vi "WriteDoubleGlobal.vi"(0 "controller in":refnum<k24>, 7 "variable number":i32, 9 "value":dbl, 11 "error in (no error)":errorcluster) -> (4 "controller out":refnum<k24>, 15 "error out":errorcluster)   [LabVIEW 2019]
uses:
  C:/Users/patrick/Documents/GitHub/Aerotech-Delay-Line/lvsrc/Aerotech-Ensemble-LabVIEW/2010-5.6/Bin/Aerotech.Ensemble.dll
  Bin/Aerotech.Ensemble.dll
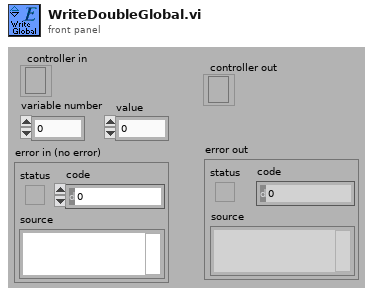
[diagram p1: front panel]
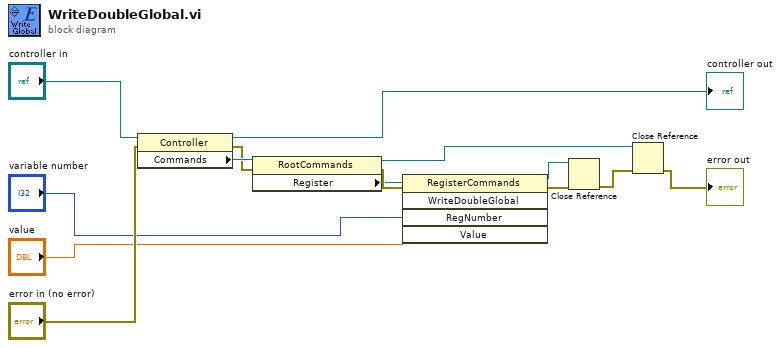
[diagram p0: block diagram]
diagram:
  n1 = property class="Controller"(reference="controller in", error in="error in (no error)") -> (reference out=→"controller out":refnum<k24>, error out=w10:errorcluster, "Commands"=w11:refnum<k24>)
  n2 = property class="RootCommands"(reference=w11, error in=w10) -> (reference out=w3:refnum<k24>, error out=w9:errorcluster, "Register"=w8:refnum<k24>)
  n3 = invoke class="RegisterCommands" method="WriteDoubleGlobal"(reference=w8, error in=w9, "RegNumber"="variable number", "Value"="value") -> (reference out=w4:refnum<k24>, error out=w7:errorcluster)  [unwired: 1 in, 3 out]
  n4 = Close Reference(reference=w4, error in (no error)=w7) -> (error out=w5:errorcluster)
  n5 = Close Reference(reference=w3, error in (no error)=w5) -> (error out=→"error out":errorcluster)
